vi "Notify Closing Status.vi"(8 "error in (no error)":errorcluster, 11 "SV Data":T1={"Status notifier"=refnum, "Write FIFO ref"=refnum, "Read FIFO ref"=refnum, "Status FIFO ref"=refnum, "Update Rate"=1, "Write Refs by Type"={"DBL Write"=[]}, "Read Refs by Type"={"DBL Read"=[]}, "WriteSize"=0, "ReadSize"=0}) -> (0 "error out":errorcluster)   [LabVIEW 2020, in "Shared Variable Interface.lvlib"]
uses:
  Shared Variable Interface.lvlib
  SV Process Configuration.ctl
  <vilib>/NI VeriStand/Custom Device Tools/Custom Device Utility Library/Custom Device Utility Library.lvlib
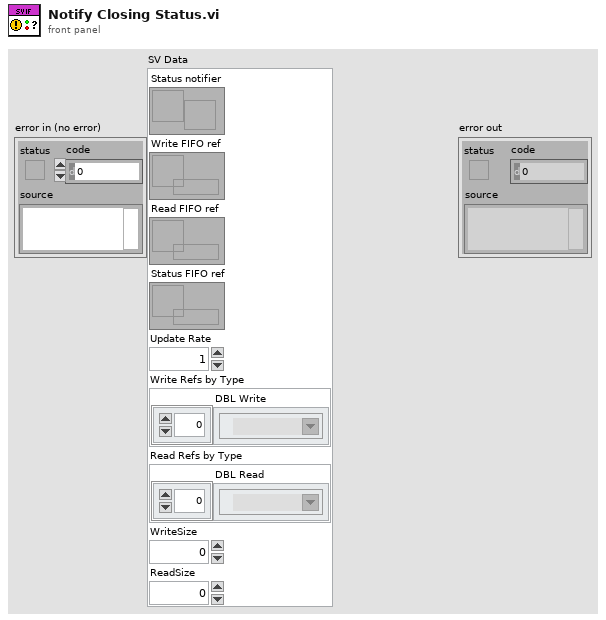
[diagram p1: front panel]
types:
  T1 = typedef "Shared Variable Interface.lvlib/SV Process Configuration.ctl" = cluster{"Status notifier":refnum<notifier>, "Write FIFO ref":refnum<k33>, "Read FIFO ref":refnum<k33>, "Status FIFO ref":refnum<k33>, "Update Rate":u32, "Write Refs by Type":cluster{"DBL Write":refnum<k21>[]}, "Read Refs by Type":cluster{"DBL Read":refnum<k21>[]}, "WriteSize":i32, "ReadSize":i32}
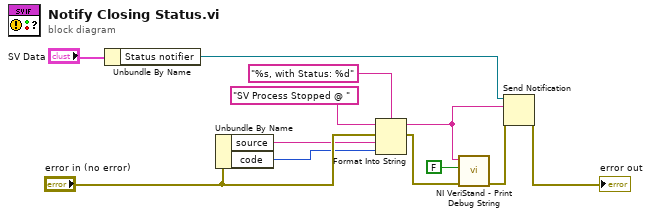
[diagram p0: block diagram]
diagram:
  n1 = Unbundle By Name("SV Data") -> ("Status notifier"=w1:refnum<notifier>)
  n2 = Unbundle By Name("error in (no error)") -> ("source"=w10:string, "code"=w9:i32)
  n3 = Format Into String(format string="%s, with Status: %d", initial string="SV Process Stopped @ " ("notification"), error in="error in (no error)", w10, w9) -> (resulting string=w7:string, error out=w3:errorcluster)
  n4 = call <vilib>:"NI VeriStand - Print Debug String.vi"("error in (no error)"=w3, "Add to log file? (F)"=FALSE ("Add to log file? (T)"), "Message"=w7) -> ("error out"=w5:errorcluster)  [unwired: 8 in]
  n5 = Send Notification(notification=w7, notifier=w1, error in (no error)=w5) -> (error out=→"error out":errorcluster)  [unwired: 1 out]
